vi "Read name.vi"(9 "SubVI in":refnum<class "SubVI.lvclass">) -> (3 "SubVI out":refnum<class "SubVI.lvclass">, 4 "name":string)   [LabVIEW 2014, in "SubVI.lvclass"]
uses:
  SubVI.lvclass
  Node/Node.lvclass
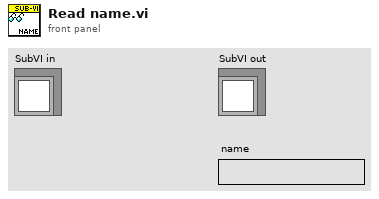
[diagram p1: front panel]
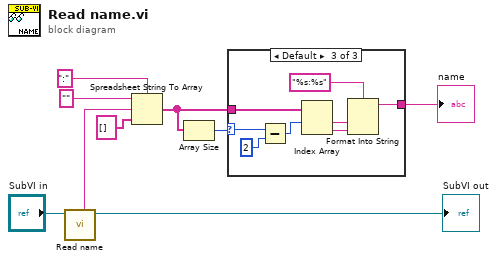
[diagram p0: block diagram]
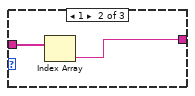
[diagram p3: hidden frame]
diagram:
  n1 = call-parent "Read name.vi"("Node in"="SubVI in") -> ("Node out"=→"SubVI out":refnum<class "SubVI.lvclass">, "name"=w7:string)  [unwired: 7 in]
  n2 = Spreadsheet String To Array(delimiter (Tab)=":", format string="", spreadsheet string=w7, array type (2D Dbl)=string[] []) -> (array=w2:string[])
  n3 = Array Size(array=w2) -> (size(s)=w3:i32)
  n4 = case shown="Default" w3 {
    selector: w3 -> [_ _ w18]
    tunnel: w2 -> [_ w11 w19]
    tunnel: [_ w10 w13] -> w1
    frame 0 {
    }
    frame 1 {
      n5 = Index Array(array=w11) -> (element=w10:string)  [unwired: 1 in]
    }
    frame Default {
      n6 = Subtract(x=w18, y=2) -> (x-y=w16:i32)
      n7 = Index Array(array=w19, index #1=w16) -> (element #1=w15:string, element #2=w14:string)  [unwired: 1 in]
      n8 = Format Into String(format string="%s:%s", w15, w14) -> (resulting string=w13:string)  [unwired: 2 in, 1 out]
    }
  }
  "name" <- w1
